vi "Create Test Node.vi"(8 "error in (no error)":errorcluster, 11 "Create Test Node Model in":refnum<class "Create Test Node Model.lvclass">) -> (0 "error out":errorcluster, 3 "Create Test Node Model out":refnum<class "Create Test Node Model.lvclass">)   [LabVIEW 2013, in "Create Test Node Model.lvlib" / "Create Test Node Model.lvclass"]
uses:
  Create Test Node Model.lvclass
  <vilib>/ActorFramework/Actor/Actor.lvclass/Actor.ctl
  Create Test Node Model.lvclass/Create Test Node Model.ctl
  <vilib>/Utility/miscctls.llb/LVPositionTypeDef.ctl
  <vilib>/ActorFrameworkMVC/UI Controller Messages/Move Subpanel Msg/Move Subpanel Msg.lvclass/Move Subpanel Msg.ctl
  <vilib>/ActorFramework/Message Enqueuer/Message Enqueuer.lvclass/Message Enqueuer.ctl
  <vilib>/ActorFrameworkMVC/UI Controller Messages/Insert Subpanel Msg/Insert Subpanel Msg.lvclass/Insert Subpanel Msg.ctl
  <vilib>/ActorFramework/Message Enqueuer/Enqueue.vi
  <vilib>/ActorFramework/Message Priority Queue/Priority Enqueue.vi
  <vilib>/ActorFrameworkMVC/UI Controller Messages/Move Subpanel Msg/Move Subpanel Msg.lvclass
  <vilib>/ActorFrameworkMVC/UI Controller Messages/Insert Subpanel Msg/Insert Subpanel Msg.lvclass
  Test Node Model Messages/Preview Test Node Msg/Preview Test Node Msg.lvclass
  Test Node Model Messages/Update Tiles Info Msg/Update Tiles Info Msg.lvclass
  Test Node Model Messages/Update Previous Button Visibility Msg/Update Previous Button Visibility Msg.lvclass
  Test Node Model Messages/Update Next Button Visibility Msg/Update Next Button Visibility Msg.lvclass
  Common/File IO/File IO.lvlib
  <vilib>/ActorFramework/Actor/Actor.lvclass
  <vilib>/ActorFrameworkMVC/UI Controller Messages/Get Model Actor Enqueuer Msg/Get Model Actor Enqueuer Msg.lvclass
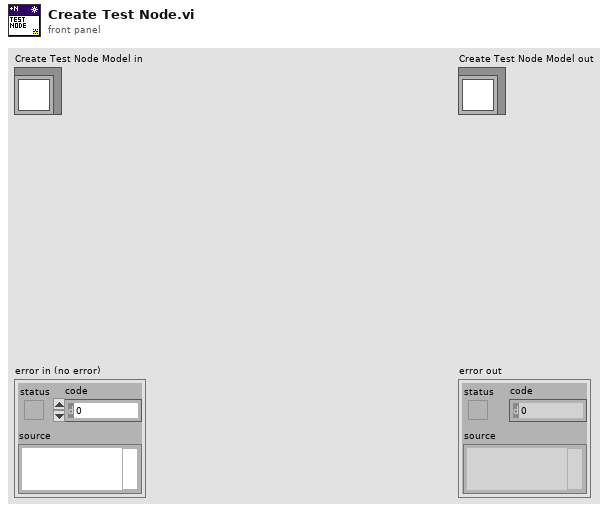
[diagram p1: front panel]
types:
  T1 = typedef "LVPositionTypeDef.ctl" = cluster{"Left":i32, "Top":i32}
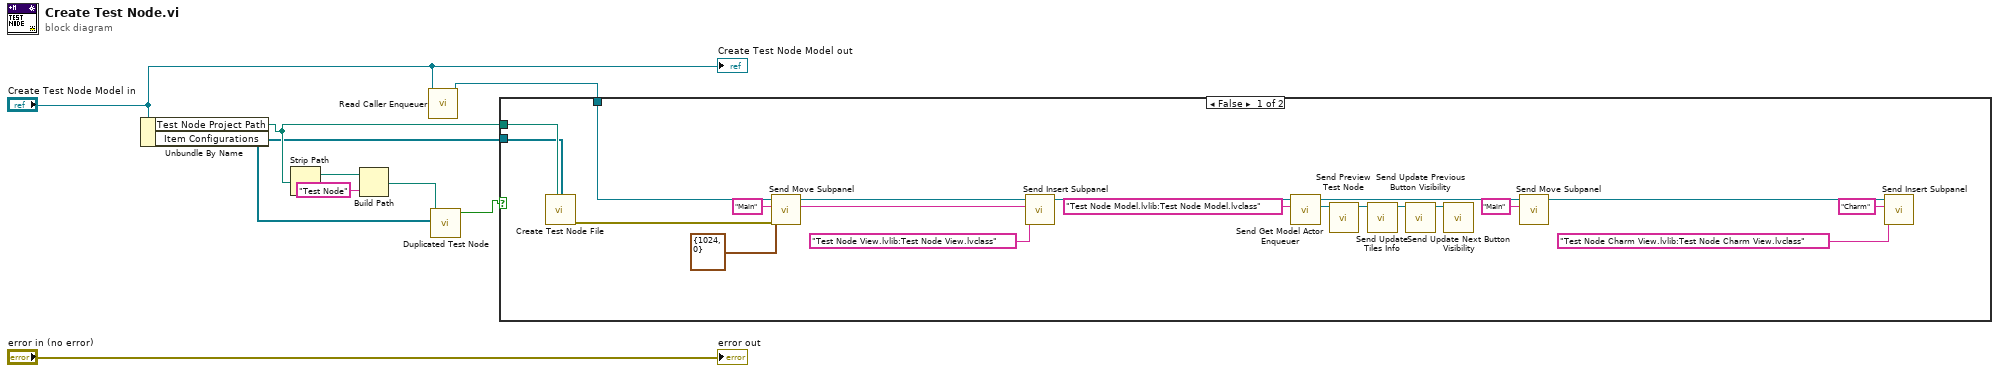
[diagram p0: block diagram]
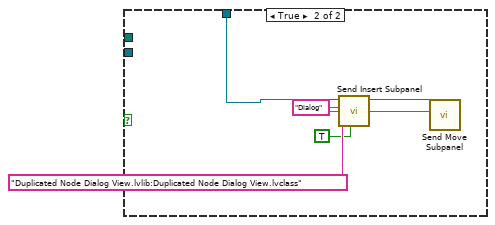
[diagram p2: hidden frame]
diagram:
  n1 = Unbundle By Name("Create Test Node Model in") -> ("Test Node Project Path"=w4:path, "Item Configurations"=w3:refnum<class "Item Configuration.lvclass">[])
  n2 = Strip Path(path=w4) -> (stripped path=w8:path)  [unwired: 1 out]
  n3 = Build Path(base path=w8, name or relative path="Test Node") -> (appended path=w6:path)
  n4 = call <vilib>:"Read Caller Enqueuer.vi"("Actor"="Create Test Node Model in") -> ("Caller Enqueuer"=w2:refnum<class "Message Enqueuer.lvclass">)  [unwired: 10 in]
  n5 = call "Duplicated Test Node.vi"("Item Configurations"=w3, "Test Node Directory Path"=w6) -> ("Duplicated?"=w5:bool)  [unwired: 9 in]
  n6 = case shown="False" w5 {
    tunnel: w4 -> [w28 _]
    tunnel: w3 -> [w27 _]
    tunnel: w2 -> [w11 w29]
    frame False {
      w23 = "Main" ("Subpanel Name")
      n7 = call "Create Test Node File.vi"("Item Configurations"=w27, "Test Node Project Path"=w28) -> ("error out"=w10:errorcluster)  [unwired: 9 in]
      n8 = call <vilib>:"Send Move Subpanel.vi"("error in (no error)"=w10, "Position (0,0)"=T1 {"Left"=1024, "Top"=0}, "Subpanel Name"=w23, "Message Enqueuer"=w11) -> ("Message Enqueuer out"=w26:refnum<class "Message Enqueuer.lvclass">)  [unwired: 6 in, 1 out]
      n9 = call <vilib>:"Send Insert Subpanel.vi"("View Name"="Test Node View.lvlib:Test Node View.lvclass" ("Subpanel Name"), "Subpanel Name"=w23, "Message Enqueuer"=w26) -> ("Message Enqueuer out"=w21:refnum<class "Message Enqueuer.lvclass">)  [unwired: 7 in, 1 out]
      n10 = call <vilib>:"Send Get Model Actor Enqueuer.vi"("Model Name"="Test Node Model.lvlib:Test Node Model.lvclass", "Message Enqueuer in"=w21) -> ("Reply"=w12:refnum<class "Message Enqueuer.lvclass">, "Message Enqueuer out"=w20:refnum<class "Message Enqueuer.lvclass">)  [unwired: 6 in, 2 out]
      n11 = call "Send Preview Test Node.vi"("Message Enqueuer"=w12) -> ("Message Enqueuer out"=w18:refnum<class "Message Enqueuer.lvclass">)  [unwired: 9 in, 1 out]
      n12 = call "Send Update Tiles Info.vi"("Message Enqueuer"=w18) -> ("Message Enqueuer out"=w17:refnum<class "Message Enqueuer.lvclass">)  [unwired: 9 in, 1 out]
      n13 = call "Send Update Previous Button Visibility.vi"("Message Enqueuer"=w17) -> ("Message Enqueuer out"=w16:refnum<class "Message Enqueuer.lvclass">)  [unwired: 9 in, 1 out]
      n14 = call "Send Update Next Button Visibility.vi"("Message Enqueuer"=w16) -> ()  [unwired: 9 in, 2 out]
      n15 = call <vilib>:"Send Move Subpanel.vi"("Subpanel Name"="Main", "Message Enqueuer"=w20) -> ("Message Enqueuer out"=w15:refnum<class "Message Enqueuer.lvclass">)  [unwired: 8 in, 1 out]
      n16 = call <vilib>:"Send Insert Subpanel.vi"("View Name"="Test Node Charm View.lvlib:Test Node Charm View.lvclass", "Subpanel Name"="Charm", "Message Enqueuer"=w15) -> ()  [unwired: 7 in, 2 out]
    }
    frame True {
      w31 = "Dialog" ("Subpanel Name")
      n17 = call <vilib>:"Send Insert Subpanel.vi"("Transparent? (F)"=TRUE, "View Name"="Duplicated Node Dialog View.lvlib:Duplicated Node Dialog View.lvclass", "Subpanel Name"=w31, "Message Enqueuer"=w29) -> ("Message Enqueuer out"=w32:refnum<class "Message Enqueuer.lvclass">)  [unwired: 6 in, 1 out]
      n18 = call <vilib>:"Send Move Subpanel.vi"("Subpanel Name"=w31, "Message Enqueuer"=w32) -> ()  [unwired: 8 in, 2 out]
    }
  }
  "error out" <- "error in (no error)"
  "Create Test Node Model out" <- "Create Test Node Model in"
